vi "GTH-V2.EEPROM.vi"(8 "Error In":errorcluster caption="错误输入", 9 "Calibration_Value_In":string[](array[string]), 10 "CMD":T1(ring), 11 "VISA资源输入":refnum<visa-resource-name>="USB0::0x3323::0x0001::48E3845A3737::RAW") -> (0 "Error Out":errorcluster caption="错误输出", 1 "Calibration_Value_Out":string[](array[string]), 3 "OK?":bool=TRUE, 4 "Return":string="05DFFF313737554343038529\r\n")   [LabVIEW 2012, in "Lib_UEL.ATE.lvlib" / "STM32-CoreBD.lvlib"]
uses:
  STM32-CoreBD.lvlib
panel:
  # "Version History\nV1.0.0,2015-8-11, 适用于新版GTH-V2硬件."
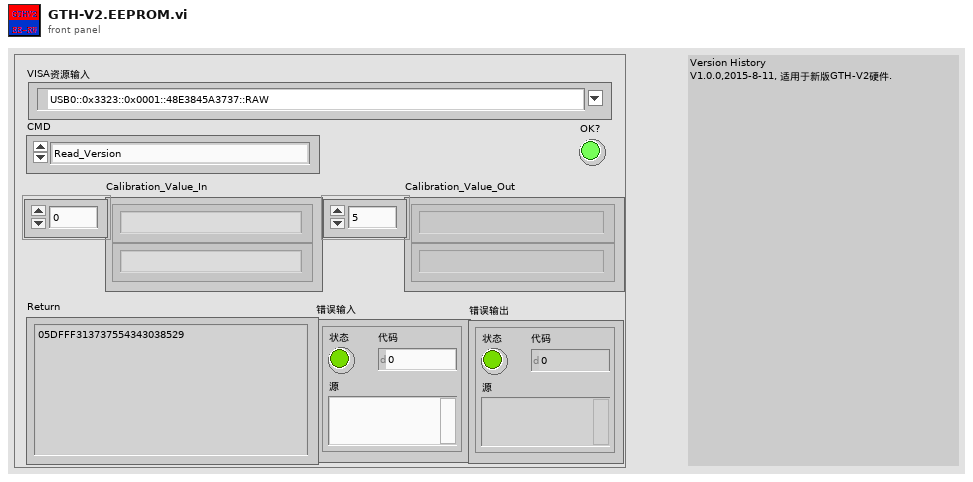
[diagram p1: front panel]
types:
  T1 = enum16{"Read_Version", "Read_PID", "Read_CalibrationInfo", "Read_C_Value_ADC_ChanA", "Read_C_Value_ADC_ChanB", "Read_C_Value_Current", "Read_C_Value_DAC", "Write_CalibrationInfo", "Write_C_Value_ADC_ChanA", "Write_C_Value_ADC_ChanB", "Write_C_Value_Current", "Write_C_Value_DAC"}
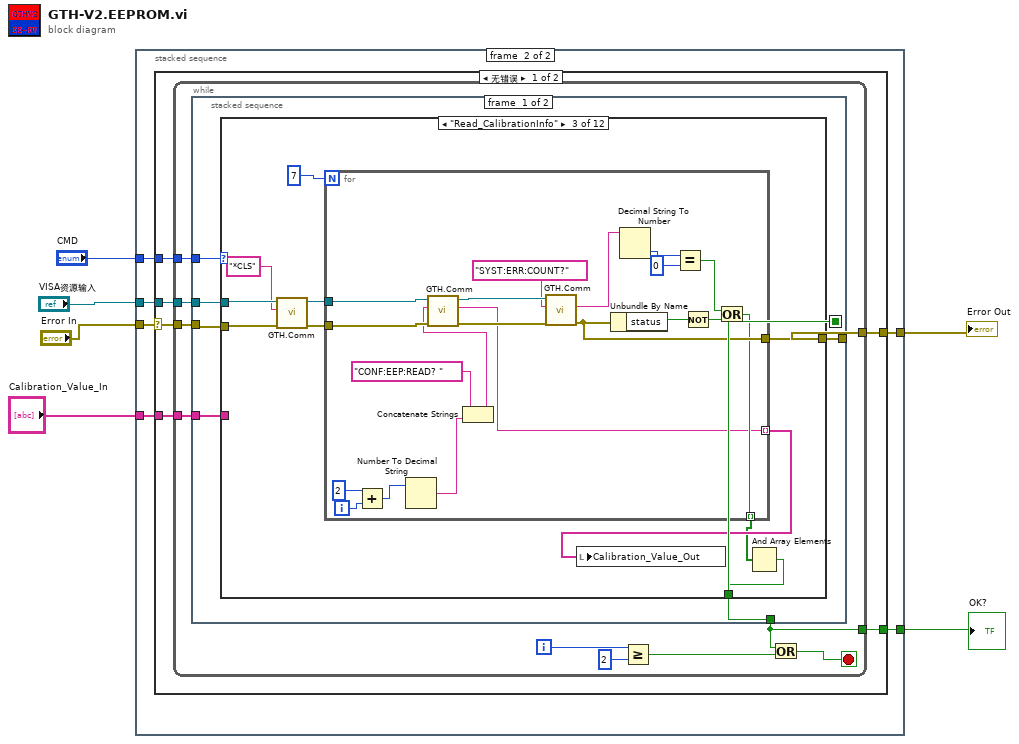
[diagram p0: block diagram]
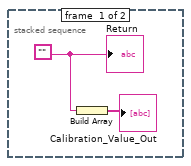
[diagram p2: hidden frame]
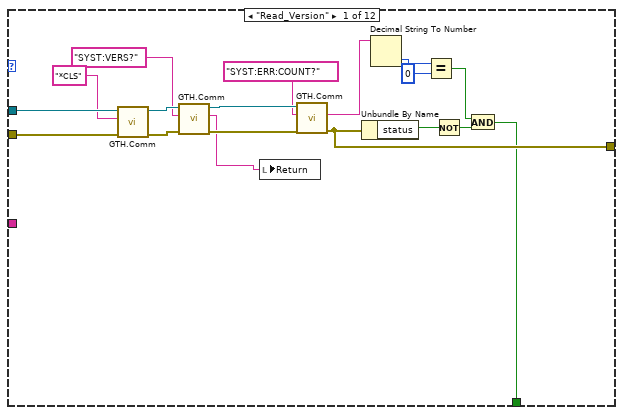
[diagram p3: hidden frame]
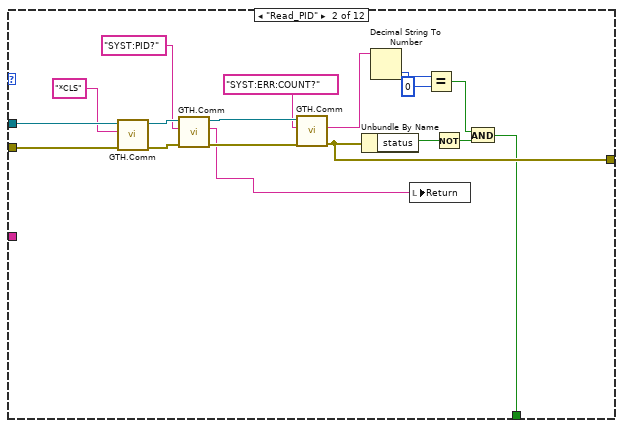
[diagram p4: hidden frame]
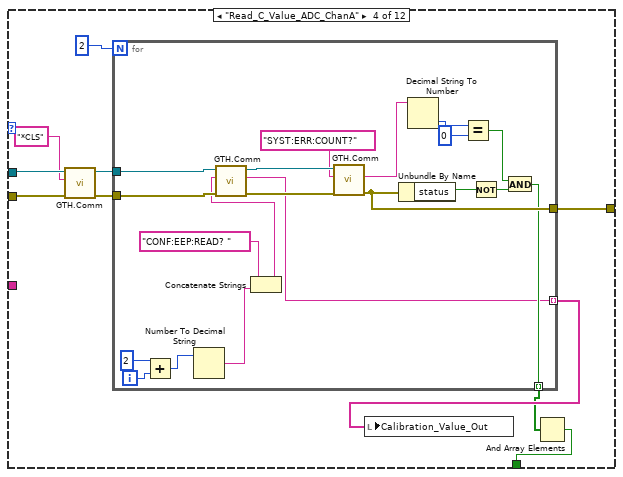
[diagram p5: hidden frame]
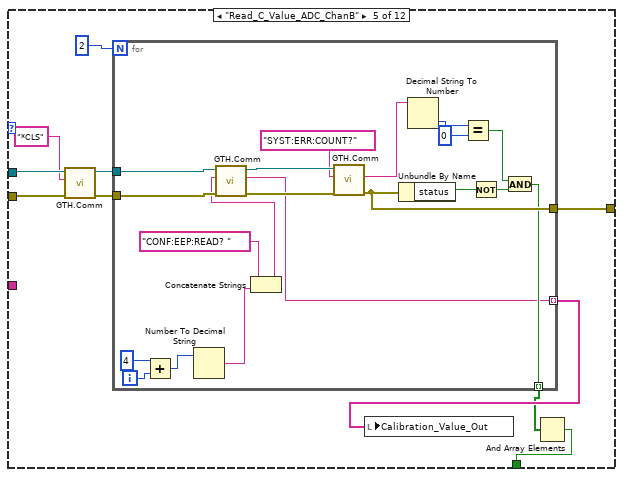
[diagram p6: hidden frame]
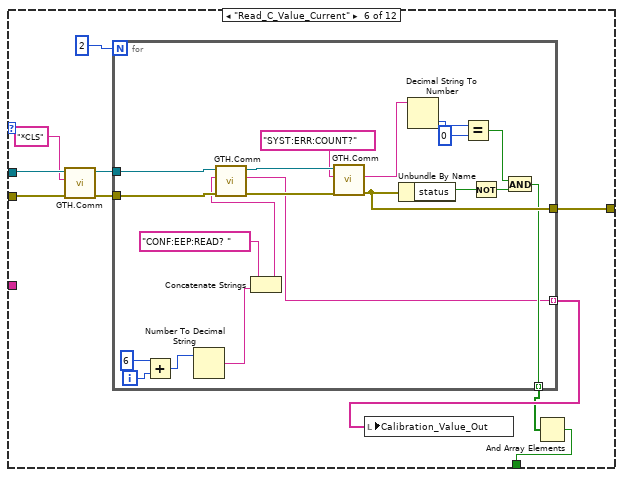
[diagram p7: hidden frame]
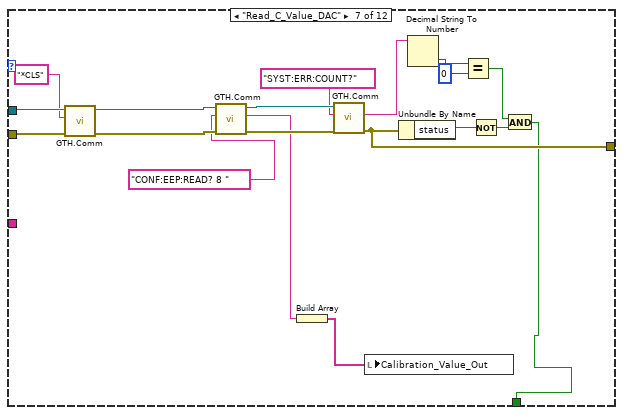
[diagram p8: hidden frame]
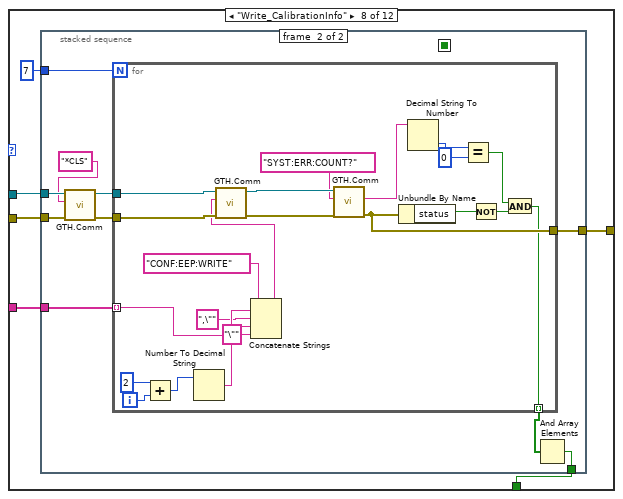
[diagram p9: hidden frame]
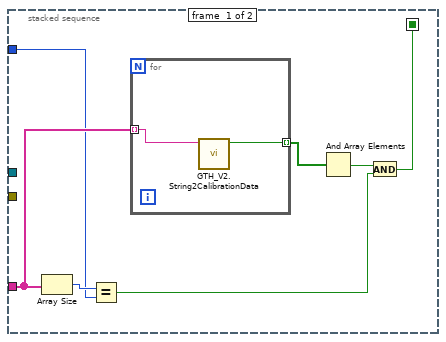
[diagram p10: hidden frame]
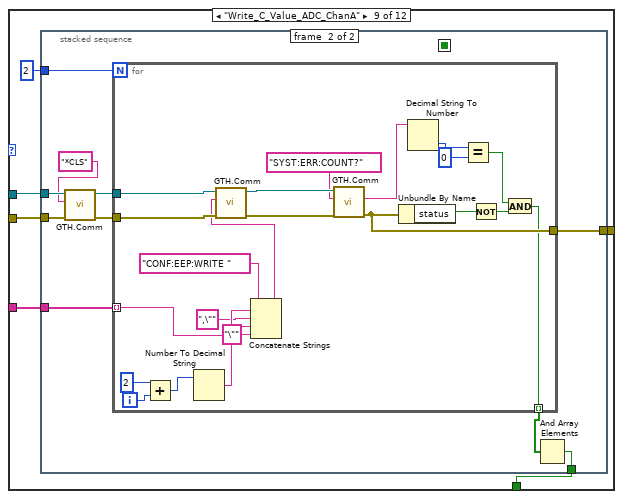
[diagram p11: hidden frame]
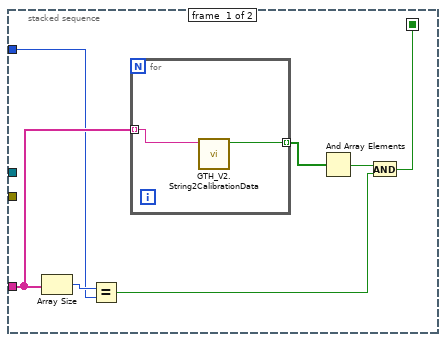
[diagram p12: hidden frame]
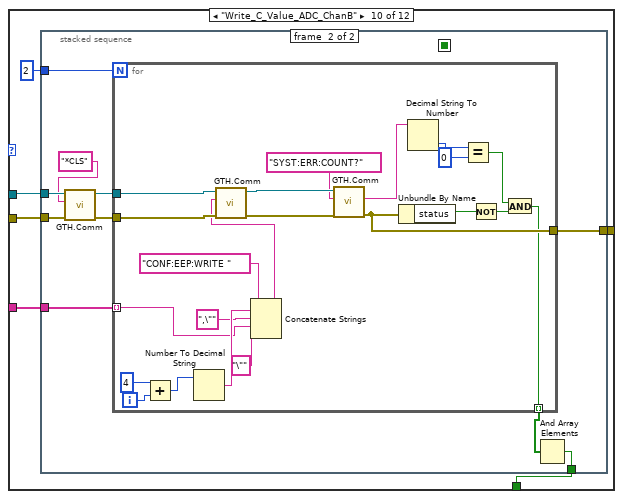
[diagram p13: hidden frame]
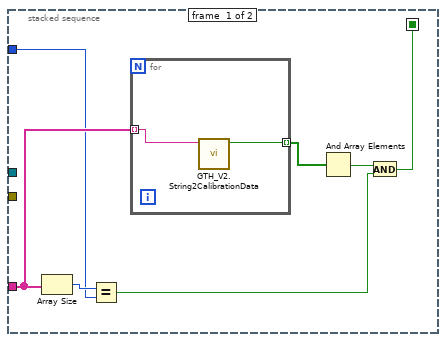
[diagram p14: hidden frame]
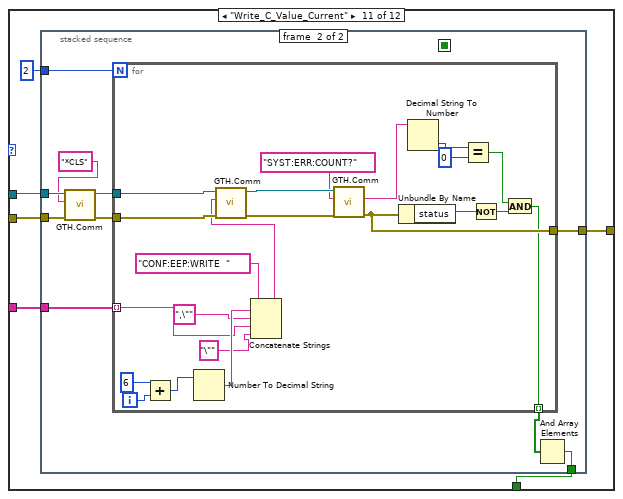
[diagram p15: hidden frame]
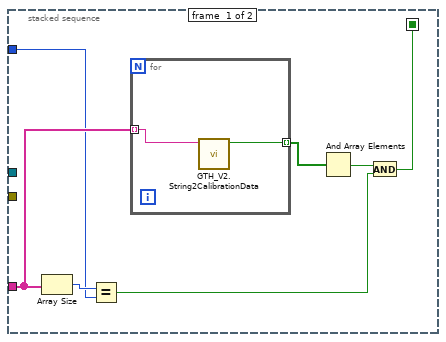
[diagram p16: hidden frame]
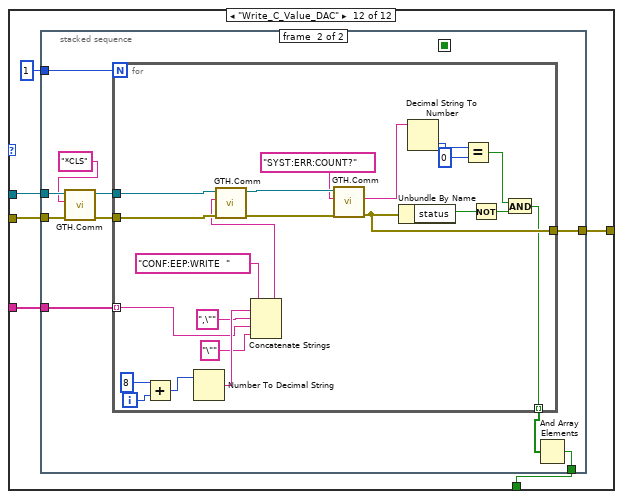
[diagram p17: hidden frame]
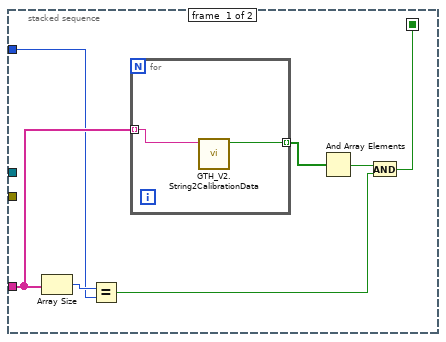
[diagram p18: hidden frame]
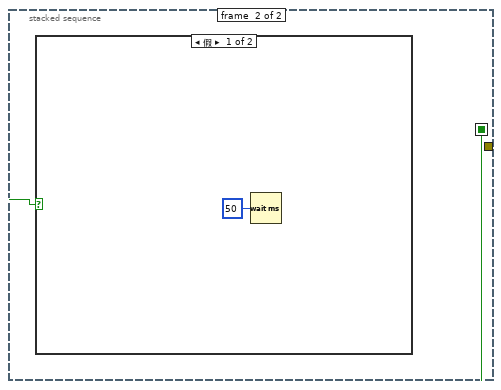
[diagram p19: hidden frame]
diagram:
  n1 = stacked-sequence {
    tunnel: "Error In" -> [_ w14]
    tunnel: "VISA资源输入" -> [_ w13]
    tunnel: [_ w12] -> w4
    tunnel: "CMD" -> [_ w11]
    tunnel: [_ w10] -> w2
    tunnel: "Calibration_Value_In" -> [_ w9]
    frame #0 {
      w8 = ""
      n2 = Build Array(w8) -> (→"Calibration_Value_Out":string[])
      "Return" <- w8
    }
    frame #1 {
      n3 = case shown="无错误" w14 {
        selector: w14 -> [w19 w449]
        tunnel: [w18 w449] -> w10
        tunnel: w13 -> [w20 _]
        tunnel: [w17 FALSE] -> w12
        tunnel: w11 -> [w16 _]
        tunnel: w9 -> [w15 _]
        frame No Error {
          n4 = while {
            tunnel: w20 -> [w30]
            tunnel: w19 -> [w29]
            tunnel: [w28] -> w18
            tunnel: [w23] -> w17
            tunnel: w16 -> [w22]
            tunnel: w15 -> [w21]
            i -> [w26]
            stop <- w27 stop-if-true
            n5 = stacked-sequence {
              seq-local: [w33 _] -> [_ w447]
              tunnel: w30 -> [w36 _]
              tunnel: w29 -> [w35 _]
              tunnel: [w34 _] -> w28
              tunnel: [w33 _] -> w23
              tunnel: w22 -> [w32 _]
              tunnel: w21 -> [w31 _]
              frame #0 {
                n6 = case shown="\"Read_CalibrationInfo\"" w32 {
                  tunnel: w36 -> [w54 w72 w82 w112 w142 w172 w211 w217 w264 w311 w358 w405]
                  tunnel: w35 -> [w53 w71 w81 w111 w141 w171 w210 w216 w263 w310 w357 w404]
                  tunnel: [w48 w66 w78 w108 w138 w168 w207 w215 w262 w309 w356 w403] -> w34
                  tunnel: [w47 w65 w73 w103 w133 w163 w193 w214 w261 w308 w355 w402] -> w33
                  tunnel: w31 -> [_ _ _ _ _ _ _ w213 w260 w307 w354 w401]
                  frame "Read_Version" {
                    n7 = call "GTH.Comm.vi"("Error In"=w53, "SCPI CMD"="*CLS", "USB Port In"=w54) -> ("Error Out"=w51:errorcluster, "USB Port Out"=w52:refnum<visa-resource-name>)  [unwired: 3 in, 4 out]
                    n8 = call "GTH.Comm.vi"("Error In"=w51, "SCPI CMD"="SYST:VERS?" ("字符串"), "USB Port In"=w52) -> ("Error Out"=w49:errorcluster, "Return"=w38:string, "USB Port Out"=w50:refnum<visa-resource-name>)  [unwired: 3 in, 3 out]
                    n9 = local write "Return"(w38) -> ()
                    n10 = call "GTH.Comm.vi"("Error In"=w49, "SCPI CMD"="SYST:ERR:COUNT?", "USB Port In"=w50) -> ("Error Out"=w48:errorcluster, "Return"=w45:string)  [unwired: 3 in, 4 out]
                    n11 = Unbundle By Name(w48) -> ("status"=w42:bool)
                    n12 = Decimal String To Number(string=w45) -> (number=w44:i32)  [unwired: 2 in, 1 out]
                    n13 = Equal?(x=w44, y=0) -> (x = y?=w40:bool)
                    n14 = Not(x=w42) -> (.not. x?=w41:bool)
                    n15 = And(x=w40, y=w41) -> (x .and. y?=w47:bool)
                  }
                  frame "Read_PID" {
                    n16 = call "GTH.Comm.vi"("Error In"=w71, "SCPI CMD"="*CLS", "USB Port In"=w72) -> ("Error Out"=w69:errorcluster, "USB Port Out"=w70:refnum<visa-resource-name>)  [unwired: 3 in, 4 out]
                    n17 = call "GTH.Comm.vi"("Error In"=w69, "SCPI CMD"="SYST:PID?" ("字符串"), "USB Port In"=w70) -> ("Error Out"=w67:errorcluster, "Return"=w56:string, "USB Port Out"=w68:refnum<visa-resource-name>)  [unwired: 3 in, 3 out]
                    n18 = call "GTH.Comm.vi"("Error In"=w67, "SCPI CMD"="SYST:ERR:COUNT?", "USB Port In"=w68) -> ("Error Out"=w66:errorcluster, "Return"=w63:string)  [unwired: 3 in, 4 out]
                    n19 = Unbundle By Name(w66) -> ("status"=w60:bool)
                    n20 = Decimal String To Number(string=w63) -> (number=w62:i32)  [unwired: 2 in, 1 out]
                    n21 = local write "Return"(w56) -> ()
                    n22 = Equal?(x=w62, y=0) -> (x = y?=w58:bool)
                    n23 = Not(x=w60) -> (.not. x?=w59:bool)
                    n24 = And(x=w58, y=w59) -> (x .and. y?=w65:bool)
                  }
                  frame "Read_CalibrationInfo" {
                    n25 = call "GTH.Comm.vi"("Error In"=w81, "SCPI CMD"="*CLS", "USB Port In"=w82) -> ("Error Out"=w79:errorcluster, "USB Port Out"=w80:refnum<visa-resource-name>)  [unwired: 3 in, 4 out]
                    n26 = for {
                      N: 7 -> [_]
                      tunnel: w80 -> [w102]
                      tunnel: w79 -> [w101]
                      tunnel: [w98] -> w78
                      tunnel: [w97] -> w74 mode=indexing
                      tunnel: [w89] -> w75 mode=indexing
                      i -> [w88]
                      n27 = Add(x=2, y=w88) -> (x+y=w86:i32)
                      n28 = Number To Decimal String(number=w86) -> (decimal integer string=w84:string)  [unwired: 1 in]
                      n29 = Concatenate Strings("CONF:EEP:READ? " ("字符串"), w84) -> (w83:string)
                      n30 = call "GTH.Comm.vi"("Error In"=w101, "SCPI CMD"=w83, "USB Port In"=w102) -> ("Error Out"=w99:errorcluster, "Return"=w89:string, "USB Port Out"=w100:refnum<visa-resource-name>)  [unwired: 3 in, 3 out]
                      n31 = call "GTH.Comm.vi"("Error In"=w99, "SCPI CMD"="SYST:ERR:COUNT?", "USB Port In"=w100) -> ("Error Out"=w98:errorcluster, "Return"=w95:string)  [unwired: 3 in, 4 out]
                      n32 = Unbundle By Name(w98) -> ("status"=w92:bool)
                      n33 = Decimal String To Number(string=w95) -> (number=w94:i32)  [unwired: 2 in, 1 out]
                      n34 = Equal?(x=w94, y=0) -> (x = y?=w90:bool)
                      n35 = Not(x=w92) -> (.not. x?=w91:bool)
                      n36 = Or(x=w90, y=w91) -> (x .or. y?=w97:bool)
                    }
                    n37 = local write "Calibration_Value_Out"(w75) -> ()
                    n38 = And Array Elements(Boolean array=w74) -> (logical AND=w73:bool)
                  }
                  frame "Read_C_Value_ADC_ChanA" {
                    n39 = call "GTH.Comm.vi"("Error In"=w111, "SCPI CMD"="*CLS", "USB Port In"=w112) -> ("Error Out"=w109:errorcluster, "USB Port Out"=w110:refnum<visa-resource-name>)  [unwired: 3 in, 4 out]
                    n40 = for {
                      N: 2 -> [_]
                      tunnel: w110 -> [w132]
                      tunnel: w109 -> [w131]
                      tunnel: [w128] -> w108
                      tunnel: [w127] -> w104 mode=indexing
                      tunnel: [w119] -> w105 mode=indexing
                      i -> [w118]
                      n41 = Add(x=2, y=w118) -> (x+y=w116:i32)
                      n42 = Number To Decimal String(number=w116) -> (decimal integer string=w114:string)  [unwired: 1 in]
                      n43 = Concatenate Strings("CONF:EEP:READ? " ("字符串"), w114) -> (w113:string)
                      n44 = call "GTH.Comm.vi"("Error In"=w131, "SCPI CMD"=w113, "USB Port In"=w132) -> ("Error Out"=w129:errorcluster, "Return"=w119:string, "USB Port Out"=w130:refnum<visa-resource-name>)  [unwired: 3 in, 3 out]
                      n45 = call "GTH.Comm.vi"("Error In"=w129, "SCPI CMD"="SYST:ERR:COUNT?", "USB Port In"=w130) -> ("Error Out"=w128:errorcluster, "Return"=w125:string)  [unwired: 3 in, 4 out]
                      n46 = Unbundle By Name(w128) -> ("status"=w122:bool)
                      n47 = Decimal String To Number(string=w125) -> (number=w124:i32)  [unwired: 2 in, 1 out]
                      n48 = Equal?(x=w124, y=0) -> (x = y?=w120:bool)
                      n49 = Not(x=w122) -> (.not. x?=w121:bool)
                      n50 = And(x=w120, y=w121) -> (x .and. y?=w127:bool)
                    }
                    n51 = local write "Calibration_Value_Out"(w105) -> ()
                    n52 = And Array Elements(Boolean array=w104) -> (logical AND=w103:bool)
                  }
                  frame "Read_C_Value_ADC_ChanB" {
                    n53 = call "GTH.Comm.vi"("Error In"=w141, "SCPI CMD"="*CLS", "USB Port In"=w142) -> ("Error Out"=w139:errorcluster, "USB Port Out"=w140:refnum<visa-resource-name>)  [unwired: 3 in, 4 out]
                    n54 = for {
                      N: 2 -> [_]
                      tunnel: w140 -> [w162]
                      tunnel: w139 -> [w161]
                      tunnel: [w158] -> w138
                      tunnel: [w157] -> w134 mode=indexing
                      tunnel: [w149] -> w135 mode=indexing
                      i -> [w148]
                      n55 = Add(x=4, y=w148) -> (x+y=w146:i32)
                      n56 = Number To Decimal String(number=w146) -> (decimal integer string=w144:string)  [unwired: 1 in]
                      n57 = Concatenate Strings("CONF:EEP:READ? " ("字符串"), w144) -> (w143:string)
                      n58 = call "GTH.Comm.vi"("Error In"=w161, "SCPI CMD"=w143, "USB Port In"=w162) -> ("Error Out"=w159:errorcluster, "Return"=w149:string, "USB Port Out"=w160:refnum<visa-resource-name>)  [unwired: 3 in, 3 out]
                      n59 = call "GTH.Comm.vi"("Error In"=w159, "SCPI CMD"="SYST:ERR:COUNT?", "USB Port In"=w160) -> ("Error Out"=w158:errorcluster, "Return"=w155:string)  [unwired: 3 in, 4 out]
                      n60 = Unbundle By Name(w158) -> ("status"=w152:bool)
                      n61 = Decimal String To Number(string=w155) -> (number=w154:i32)  [unwired: 2 in, 1 out]
                      n62 = Equal?(x=w154, y=0) -> (x = y?=w150:bool)
                      n63 = Not(x=w152) -> (.not. x?=w151:bool)
                      n64 = And(x=w150, y=w151) -> (x .and. y?=w157:bool)
                    }
                    n65 = local write "Calibration_Value_Out"(w135) -> ()
                    n66 = And Array Elements(Boolean array=w134) -> (logical AND=w133:bool)
                  }
                  frame "Read_C_Value_Current" {
                    n67 = call "GTH.Comm.vi"("Error In"=w171, "SCPI CMD"="*CLS", "USB Port In"=w172) -> ("Error Out"=w169:errorcluster, "USB Port Out"=w170:refnum<visa-resource-name>)  [unwired: 3 in, 4 out]
                    n68 = for {
                      N: 2 -> [_]
                      tunnel: w170 -> [w192]
                      tunnel: w169 -> [w191]
                      tunnel: [w188] -> w168
                      tunnel: [w187] -> w164 mode=indexing
                      tunnel: [w179] -> w165 mode=indexing
                      i -> [w178]
                      n69 = Add(x=6, y=w178) -> (x+y=w176:i32)
                      n70 = Number To Decimal String(number=w176) -> (decimal integer string=w174:string)  [unwired: 1 in]
                      n71 = Concatenate Strings("CONF:EEP:READ? " ("字符串"), w174) -> (w173:string)
                      n72 = call "GTH.Comm.vi"("Error In"=w191, "SCPI CMD"=w173, "USB Port In"=w192) -> ("Error Out"=w189:errorcluster, "Return"=w179:string, "USB Port Out"=w190:refnum<visa-resource-name>)  [unwired: 3 in, 3 out]
                      n73 = call "GTH.Comm.vi"("Error In"=w189, "SCPI CMD"="SYST:ERR:COUNT?", "USB Port In"=w190) -> ("Error Out"=w188:errorcluster, "Return"=w185:string)  [unwired: 3 in, 4 out]
                      n74 = Unbundle By Name(w188) -> ("status"=w182:bool)
                      n75 = Decimal String To Number(string=w185) -> (number=w184:i32)  [unwired: 2 in, 1 out]
                      n76 = Equal?(x=w184, y=0) -> (x = y?=w180:bool)
                      n77 = Not(x=w182) -> (.not. x?=w181:bool)
                      n78 = And(x=w180, y=w181) -> (x .and. y?=w187:bool)
                    }
                    n79 = local write "Calibration_Value_Out"(w165) -> ()
                    n80 = And Array Elements(Boolean array=w164) -> (logical AND=w163:bool)
                  }
                  frame "Read_C_Value_DAC" {
                    n81 = call "GTH.Comm.vi"("Error In"=w210, "SCPI CMD"="*CLS", "USB Port In"=w211) -> ("Error Out"=w208:errorcluster, "USB Port Out"=w209:refnum<visa-resource-name>)  [unwired: 3 in, 4 out]
                    n82 = call "GTH.Comm.vi"("Error In"=w208, "SCPI CMD"="CONF:EEP:READ? 8 " ("字符串"), "USB Port In"=w209) -> ("Error Out"=w204:errorcluster, "Return"=w195:string, "USB Port Out"=w205:refnum<visa-resource-name>)  [unwired: 3 in, 3 out]
                    n83 = Build Array(w195) -> (w194:string[])
                    n84 = call "GTH.Comm.vi"("Error In"=w204, "SCPI CMD"="SYST:ERR:COUNT?", "USB Port In"=w205) -> ("Error Out"=w207:errorcluster, "Return"=w202:string)  [unwired: 3 in, 4 out]
                    n85 = local write "Calibration_Value_Out"(w194) -> ()
                    n86 = Unbundle By Name(w207) -> ("status"=w199:bool)
                    n87 = Decimal String To Number(string=w202) -> (number=w201:i32)  [unwired: 2 in, 1 out]
                    n88 = Equal?(x=w201, y=0) -> (x = y?=w197:bool)
                    n89 = Not(x=w199) -> (.not. x?=w198:bool)
                    n90 = And(x=w197, y=w198) -> (x .and. y?=w193:bool)
                  }
                  frame "Write_CalibrationInfo" {
                    n91 = stacked-sequence {
                      seq-local: [w219 _] -> [_ _]
                      tunnel: w217 -> [_ w236]
                      tunnel: w216 -> [_ w235]
                      tunnel: [_ w232] -> w215
                      tunnel: [_ w229] -> w214
                      tunnel: w213 -> [w223 w228]
                      tunnel: 7 -> [w218 w227]
                      frame #0 {
                        n92 = Array Size(array=w223) -> (size(s)=w224:i32)
                        n93 = Equal?(x=w224, y=w218) -> (x = y?=w220:bool)
                        n94 = for {
                          tunnel: w223 -> [w226] mode=indexing
                          tunnel: [w225] -> w222 mode=indexing
                          n95 = call "GTH_V2.String2CalibrationData.vi"("String"=w226) -> ("OK?"=w225:bool)  [unwired: 5 in, 5 out]
                        }
                        n96 = And Array Elements(Boolean array=w222) -> (logical AND=w221:bool)
                        n97 = And(x=w221, y=w220) -> (x .and. y?=w219:bool)
                      }
                      frame #1 {
                        n98 = call "GTH.Comm.vi"("Error In"=w235, "SCPI CMD"="*CLS", "USB Port In"=w236) -> ("Error Out"=w233:errorcluster, "USB Port Out"=w234:refnum<visa-resource-name>)  [unwired: 3 in, 4 out]
                        n99 = for {
                          N: w227 -> [_]
                          tunnel: w234 -> [w258]
                          tunnel: w233 -> [w257]
                          tunnel: [w254] -> w232
                          tunnel: [w253] -> w230 mode=indexing
                          tunnel: w228 -> [w238] mode=indexing
                          i -> [w245]
                          n100 = Add(x=2, y=w245) -> (x+y=w243:i32)
                          n101 = Number To Decimal String(number=w243) -> (decimal integer string=w241:string)  [unwired: 1 in]
                          n102 = Concatenate Strings("CONF:EEP:WRITE" ("字符串"), w241, ",\"" ("字符串"), w238, "\"" ("字符串")) -> (w240:string)
                          n103 = call "GTH.Comm.vi"("Error In"=w257, "SCPI CMD"=w240, "USB Port In"=w258) -> ("Error Out"=w255:errorcluster, "USB Port Out"=w256:refnum<visa-resource-name>)  [unwired: 3 in, 4 out]
                          n104 = call "GTH.Comm.vi"("Error In"=w255, "SCPI CMD"="SYST:ERR:COUNT?", "USB Port In"=w256) -> ("Error Out"=w254:errorcluster, "Return"=w251:string)  [unwired: 3 in, 4 out]
                          n105 = Unbundle By Name(w254) -> ("status"=w248:bool)
                          n106 = Decimal String To Number(string=w251) -> (number=w250:i32)  [unwired: 2 in, 1 out]
                          n107 = Equal?(x=w250, y=0) -> (x = y?=w246:bool)
                          n108 = Not(x=w248) -> (.not. x?=w247:bool)
                          n109 = And(x=w246, y=w247) -> (x .and. y?=w253:bool)
                        }
                        n110 = And Array Elements(Boolean array=w230) -> (logical AND=w229:bool)
                      }
                    }
                  }
                  frame "Write_C_Value_ADC_ChanA" {
                    n111 = stacked-sequence {
                      seq-local: [w266 _] -> [_ _]
                      tunnel: w264 -> [_ w283]
                      tunnel: w263 -> [_ w282]
                      tunnel: [_ w279] -> w262
                      tunnel: [_ w276] -> w261
                      tunnel: w260 -> [w270 w275]
                      tunnel: 2 -> [w265 w274]
                      frame #0 {
                        n112 = Array Size(array=w270) -> (size(s)=w271:i32)
                        n113 = Equal?(x=w271, y=w265) -> (x = y?=w267:bool)
                        n114 = for {
                          tunnel: w270 -> [w273] mode=indexing
                          tunnel: [w272] -> w269 mode=indexing
                          n115 = call "GTH_V2.String2CalibrationData.vi"("String"=w273) -> ("OK?"=w272:bool)  [unwired: 5 in, 5 out]
                        }
                        n116 = And Array Elements(Boolean array=w269) -> (logical AND=w268:bool)
                        n117 = And(x=w268, y=w267) -> (x .and. y?=w266:bool)
                      }
                      frame #1 {
                        n118 = call "GTH.Comm.vi"("Error In"=w282, "SCPI CMD"="*CLS", "USB Port In"=w283) -> ("Error Out"=w280:errorcluster, "USB Port Out"=w281:refnum<visa-resource-name>)  [unwired: 3 in, 4 out]
                        n119 = for {
                          N: w274 -> [_]
                          tunnel: w281 -> [w305]
                          tunnel: w280 -> [w304]
                          tunnel: [w301] -> w279
                          tunnel: [w300] -> w277 mode=indexing
                          tunnel: w275 -> [w285] mode=indexing
                          i -> [w292]
                          n120 = Add(x=2, y=w292) -> (x+y=w290:i32)
                          n121 = Number To Decimal String(number=w290) -> (decimal integer string=w288:string)  [unwired: 1 in]
                          n122 = Concatenate Strings("CONF:EEP:WRITE " ("字符串"), w288, ",\"" ("字符串"), w285, "\"" ("字符串")) -> (w287:string)
                          n123 = call "GTH.Comm.vi"("Error In"=w304, "SCPI CMD"=w287, "USB Port In"=w305) -> ("Error Out"=w302:errorcluster, "USB Port Out"=w303:refnum<visa-resource-name>)  [unwired: 3 in, 4 out]
                          n124 = call "GTH.Comm.vi"("Error In"=w302, "SCPI CMD"="SYST:ERR:COUNT?", "USB Port In"=w303) -> ("Error Out"=w301:errorcluster, "Return"=w298:string)  [unwired: 3 in, 4 out]
                          n125 = Unbundle By Name(w301) -> ("status"=w295:bool)
                          n126 = Decimal String To Number(string=w298) -> (number=w297:i32)  [unwired: 2 in, 1 out]
                          n127 = Equal?(x=w297, y=0) -> (x = y?=w293:bool)
                          n128 = Not(x=w295) -> (.not. x?=w294:bool)
                          n129 = And(x=w293, y=w294) -> (x .and. y?=w300:bool)
                        }
                        n130 = And Array Elements(Boolean array=w277) -> (logical AND=w276:bool)
                      }
                    }
                  }
                  frame "Write_C_Value_ADC_ChanB" {
                    n131 = stacked-sequence {
                      seq-local: [w313 _] -> [_ _]
                      tunnel: w311 -> [_ w330]
                      tunnel: w310 -> [_ w329]
                      tunnel: [_ w326] -> w309
                      tunnel: [_ w323] -> w308
                      tunnel: w307 -> [w317 w322]
                      tunnel: 2 -> [w312 w321]
                      frame #0 {
                        n132 = Array Size(array=w317) -> (size(s)=w318:i32)
                        n133 = Equal?(x=w318, y=w312) -> (x = y?=w314:bool)
                        n134 = for {
                          tunnel: w317 -> [w320] mode=indexing
                          tunnel: [w319] -> w316 mode=indexing
                          n135 = call "GTH_V2.String2CalibrationData.vi"("String"=w320) -> ("OK?"=w319:bool)  [unwired: 5 in, 5 out]
                        }
                        n136 = And Array Elements(Boolean array=w316) -> (logical AND=w315:bool)
                        n137 = And(x=w315, y=w314) -> (x .and. y?=w313:bool)
                      }
                      frame #1 {
                        n138 = call "GTH.Comm.vi"("Error In"=w329, "SCPI CMD"="*CLS", "USB Port In"=w330) -> ("Error Out"=w327:errorcluster, "USB Port Out"=w328:refnum<visa-resource-name>)  [unwired: 3 in, 4 out]
                        n139 = for {
                          N: w321 -> [_]
                          tunnel: w328 -> [w352]
                          tunnel: w327 -> [w351]
                          tunnel: [w348] -> w326
                          tunnel: [w347] -> w324 mode=indexing
                          tunnel: w322 -> [w332] mode=indexing
                          i -> [w339]
                          n140 = Add(x=4, y=w339) -> (x+y=w337:i32)
                          n141 = Number To Decimal String(number=w337) -> (decimal integer string=w335:string)  [unwired: 1 in]
                          n142 = Concatenate Strings("CONF:EEP:WRITE " ("字符串"), w335, ",\"" ("字符串"), w332, "\"" ("字符串")) -> (w334:string)
                          n143 = call "GTH.Comm.vi"("Error In"=w351, "SCPI CMD"=w334, "USB Port In"=w352) -> ("Error Out"=w349:errorcluster, "USB Port Out"=w350:refnum<visa-resource-name>)  [unwired: 3 in, 4 out]
                          n144 = call "GTH.Comm.vi"("Error In"=w349, "SCPI CMD"="SYST:ERR:COUNT?", "USB Port In"=w350) -> ("Error Out"=w348:errorcluster, "Return"=w345:string)  [unwired: 3 in, 4 out]
                          n145 = Unbundle By Name(w348) -> ("status"=w342:bool)
                          n146 = Decimal String To Number(string=w345) -> (number=w344:i32)  [unwired: 2 in, 1 out]
                          n147 = Equal?(x=w344, y=0) -> (x = y?=w340:bool)
                          n148 = Not(x=w342) -> (.not. x?=w341:bool)
                          n149 = And(x=w340, y=w341) -> (x .and. y?=w347:bool)
                        }
                        n150 = And Array Elements(Boolean array=w324) -> (logical AND=w323:bool)
                      }
                    }
                  }
                  frame "Write_C_Value_Current" {
                    n151 = stacked-sequence {
                      seq-local: [w360 _] -> [_ _]
                      tunnel: w358 -> [_ w377]
                      tunnel: w357 -> [_ w376]
                      tunnel: [_ w373] -> w356
                      tunnel: [_ w370] -> w355
                      tunnel: w354 -> [w364 w369]
                      tunnel: 2 -> [w359 w368]
                      frame #0 {
                        n152 = Array Size(array=w364) -> (size(s)=w365:i32)
                        n153 = Equal?(x=w365, y=w359) -> (x = y?=w361:bool)
                        n154 = for {
                          tunnel: w364 -> [w367] mode=indexing
                          tunnel: [w366] -> w363 mode=indexing
                          n155 = call "GTH_V2.String2CalibrationData.vi"("String"=w367) -> ("OK?"=w366:bool)  [unwired: 5 in, 5 out]
                        }
                        n156 = And Array Elements(Boolean array=w363) -> (logical AND=w362:bool)
                        n157 = And(x=w362, y=w361) -> (x .and. y?=w360:bool)
                      }
                      frame #1 {
                        n158 = call "GTH.Comm.vi"("Error In"=w376, "SCPI CMD"="*CLS", "USB Port In"=w377) -> ("Error Out"=w374:errorcluster, "USB Port Out"=w375:refnum<visa-resource-name>)  [unwired: 3 in, 4 out]
                        n159 = for {
                          N: w368 -> [_]
                          tunnel: w375 -> [w399]
                          tunnel: w374 -> [w398]
                          tunnel: [w395] -> w373
                          tunnel: [w394] -> w371 mode=indexing
                          tunnel: w369 -> [w380] mode=indexing
                          i -> [w386]
                          n160 = Add(x=6, y=w386) -> (x+y=w384:i32)
                          n161 = Number To Decimal String(number=w384) -> (decimal integer string=w382:string)  [unwired: 1 in]
                          n162 = Concatenate Strings("CONF:EEP:WRITE  " ("字符串"), w382, ",\"" ("字符串"), w380, "\"" ("字符串")) -> (w381:string)
                          n163 = call "GTH.Comm.vi"("Error In"=w398, "SCPI CMD"=w381, "USB Port In"=w399) -> ("Error Out"=w396:errorcluster, "USB Port Out"=w397:refnum<visa-resource-name>)  [unwired: 3 in, 4 out]
                          n164 = call "GTH.Comm.vi"("Error In"=w396, "SCPI CMD"="SYST:ERR:COUNT?", "USB Port In"=w397) -> ("Error Out"=w395:errorcluster, "Return"=w392:string)  [unwired: 3 in, 4 out]
                          n165 = Unbundle By Name(w395) -> ("status"=w389:bool)
                          n166 = Decimal String To Number(string=w392) -> (number=w391:i32)  [unwired: 2 in, 1 out]
                          n167 = Equal?(x=w391, y=0) -> (x = y?=w387:bool)
                          n168 = Not(x=w389) -> (.not. x?=w388:bool)
                          n169 = And(x=w387, y=w388) -> (x .and. y?=w394:bool)
                        }
                        n170 = And Array Elements(Boolean array=w371) -> (logical AND=w370:bool)
                      }
                    }
                  }
                  frame "Write_C_Value_DAC" {
                    n171 = stacked-sequence {
                      seq-local: [w407 _] -> [_ _]
                      tunnel: w405 -> [_ w424]
                      tunnel: w404 -> [_ w423]
                      tunnel: [_ w420] -> w403
                      tunnel: [_ w417] -> w402
                      tunnel: w401 -> [w411 w416]
                      tunnel: 1 -> [w406 w415]
                      frame #0 {
                        n172 = Array Size(array=w411) -> (size(s)=w412:i32)
                        n173 = Equal?(x=w412, y=w406) -> (x = y?=w408:bool)
                        n174 = for {
                          tunnel: w411 -> [w414] mode=indexing
                          tunnel: [w413] -> w410 mode=indexing
                          n175 = call "GTH_V2.String2CalibrationData.vi"("String"=w414) -> ("OK?"=w413:bool)  [unwired: 5 in, 5 out]
                        }
                        n176 = And Array Elements(Boolean array=w410) -> (logical AND=w409:bool)
                        n177 = And(x=w409, y=w408) -> (x .and. y?=w407:bool)
                      }
                      frame #1 {
                        n178 = call "GTH.Comm.vi"("Error In"=w423, "SCPI CMD"="*CLS", "USB Port In"=w424) -> ("Error Out"=w421:errorcluster, "USB Port Out"=w422:refnum<visa-resource-name>)  [unwired: 3 in, 4 out]
                        n179 = for {
                          N: w415 -> [_]
                          tunnel: w422 -> [w446]
                          tunnel: w421 -> [w445]
                          tunnel: [w442] -> w420
                          tunnel: [w441] -> w418 mode=indexing
                          tunnel: w416 -> [w426] mode=indexing
                          i -> [w433]
                          n180 = Add(x=8, y=w433) -> (x+y=w431:i32)
                          n181 = Number To Decimal String(number=w431) -> (decimal integer string=w429:string)  [unwired: 1 in]
                          n182 = Concatenate Strings("CONF:EEP:WRITE  " ("字符串"), w429, ",\"" ("字符串"), w426, "\"" ("字符串")) -> (w428:string)
                          n183 = call "GTH.Comm.vi"("Error In"=w445, "SCPI CMD"=w428, "USB Port In"=w446) -> ("Error Out"=w443:errorcluster, "USB Port Out"=w444:refnum<visa-resource-name>)  [unwired: 3 in, 4 out]
                          n184 = call "GTH.Comm.vi"("Error In"=w443, "SCPI CMD"="SYST:ERR:COUNT?", "USB Port In"=w444) -> ("Error Out"=w442:errorcluster, "Return"=w439:string)  [unwired: 3 in, 4 out]
                          n185 = Unbundle By Name(w442) -> ("status"=w436:bool)
                          n186 = Decimal String To Number(string=w439) -> (number=w438:i32)  [unwired: 2 in, 1 out]
                          n187 = Equal?(x=w438, y=0) -> (x = y?=w434:bool)
                          n188 = Not(x=w436) -> (.not. x?=w435:bool)
                          n189 = And(x=w434, y=w435) -> (x .and. y?=w441:bool)
                        }
                        n190 = And Array Elements(Boolean array=w418) -> (logical AND=w417:bool)
                      }
                    }
                  }
                }
              }
              frame #1 {
                n191 = case shown="假" w447 {
                  frame False {
                    n192 = Wait (ms)(milliseconds to wait=u32 50 ("等待时间（毫秒）")) -> ()  [unwired: 1 out]
                  }
                  frame True {
                  }
                }
              }
            }
            n193 = Greater Or Equal?(x=w26, y=2) -> (x >= y?=w24:bool)
            n194 = Or(x=w23, y=w24) -> (x .or. y?=w27:bool)
          }
        }
        frame Error {
          (unwired) string[] []
        }
      }
    }
  }
  "Error Out" <- w2
  "OK?" <- w4
